vi "Get Data String.vi"(8 "error in (no error)":errorcluster, 11 "Data Cluster Out":T1 {"VestaTemperature"."Water Heater Temp (°F)" min=32 max=203}) -> (0 "error out":errorcluster, 3 "Data Cluster Output":T1={"Vesta Data Output"={"Temp_W_Raw_U"=0, "Temp_W_Raw_L"=0, "Temperature Water (F)"=0.0, "Temperature Water Compensated (F)"=0.0, "Temperature Ambient (F)"=0.0, "Setpoint Location (F)"=0.0, "Heat Request"="", "Fault Ram"="", "PWM DCDC Value"=0, "Pilot Voltage (mV)"=0.0, "Setpoint Actual (F)"=0.0, "Differential Actual (F)"=0.0, "Setpoint User (F)"=0.0, "Differential User (F)"=0.0, "Termperature FIltered -TCO (F)"=0.0, "Temp_C_Raw_1 - Sensor Voltage"="", "Temp_C_Raw_2 - Sensor Voltage"="", "Chamber Sensor Temperature (F)"=0.0, "LDO Base Temperature (F)"=0.0, "LDO Timer (sec)"=0, "Disabled (0)"=FALSE, "Warming (1)"=FALSE, "Heating (2)"=FALSE, "Cooling Data Write (3)"=FALSE, "Cooling (4)"=FALSE, "Data Read (5)"=FALSE, "N/A"=FALSE, "Temperature Trip (7)"=FALSE, "Burner"=FALSE}, "VestaTemperature"={"Water Heater Temp (°F)"=135, "Differential  (°F)"=10.0}, "Timer Application Data"={"Duty Cycle"={"Burner ON Time (Seconds)"=60.0, "Burner OFF Time (Seconds)"=60.0, "Main Burner Flag"=FALSE, "Burner Power Mode"=0}}, "Data Array"=[], "MW Output"={"TC1-Channel 021"=0.0, "TC2-Channel 022"=0.0, "TC3-Channel 023"=0.0, "TC4-Channel 024"=0.0, "TC5-Channel 025"=0.0, "TC6-Channel 026"=0.0, "TC7-Channel 017"=0.0, "TC8-Channel 028"=0.0, "TC9-Channel 029"=0.0, "TC10-Channel 030"=0.0, "TC Tree Average"=0.0, "TC DWN- Channel 027"=0.0, "RTDin-Channel 031"=0.0, "RTDout-Channel 032"=0.0, "RTDamb-Channel 033"=0.0, "PSI1-Channel 011"=0.0, "PSI2-Channel 012"=0.0, "PSI3-Channel 013"=0.0, "PSI4-Channel 014"=0.0, "UE State-Channel 015"=0.0, "LE State-Channel 016"=0.0, "Module 4 Relay Status Output"={"INTELLIFAUCET TEMP(T)/FLOW(F) (CH 041)"=FALSE, "INTELLIFAUCET READY (CH 042)"=FALSE, "INTELLIFAUCET START (CH 043)"=FALSE, "INTELLIFAUCET STOP (CH 044)"=FALSE, "MAIN POWER RELAY (CH 047)"=FALSE, "NOT USED (CH 045)"=FALSE, "NOT USED (CH 046)"=FALSE, "PURGE VALVE RELAY (CH 048)"=FALSE, "OUTLET VALVE RELAY (CH 049)"=FALSE, "INLET VALVE RELAY (CH 050)"=FALSE, "Intellifaucet (% Open)"=0.0, "Proportioning Valve (%Open)"=0.0, "Intellifaucet Temp Setpoint (F)"=0.0}}} {"VestaTemperature"."Water Heater Temp (°F)" min=32 max=203})   [LabVIEW 2023]
uses:
  controls/UI Data.ctl
  Drivers/Resideo Gas Valve/Type Definitions/Vesta Info.ctl
  Drivers/Resideo Gas Valve/Type Definitions/Temperature Control.ctl
  controls/Timer Application Cluster.ctl
  controls/Burner Duty Cycle.ctl
  Hybrid Water Heater/Type Definitions/HEWH MW100 Data Cluster.ctl
  Hybrid Water Heater/Custom Instrument Control/MW100/Type Definitions/HEWH Module 4 Relay Status.ctl
panel:
  out "Data Array":string[][](array[string])
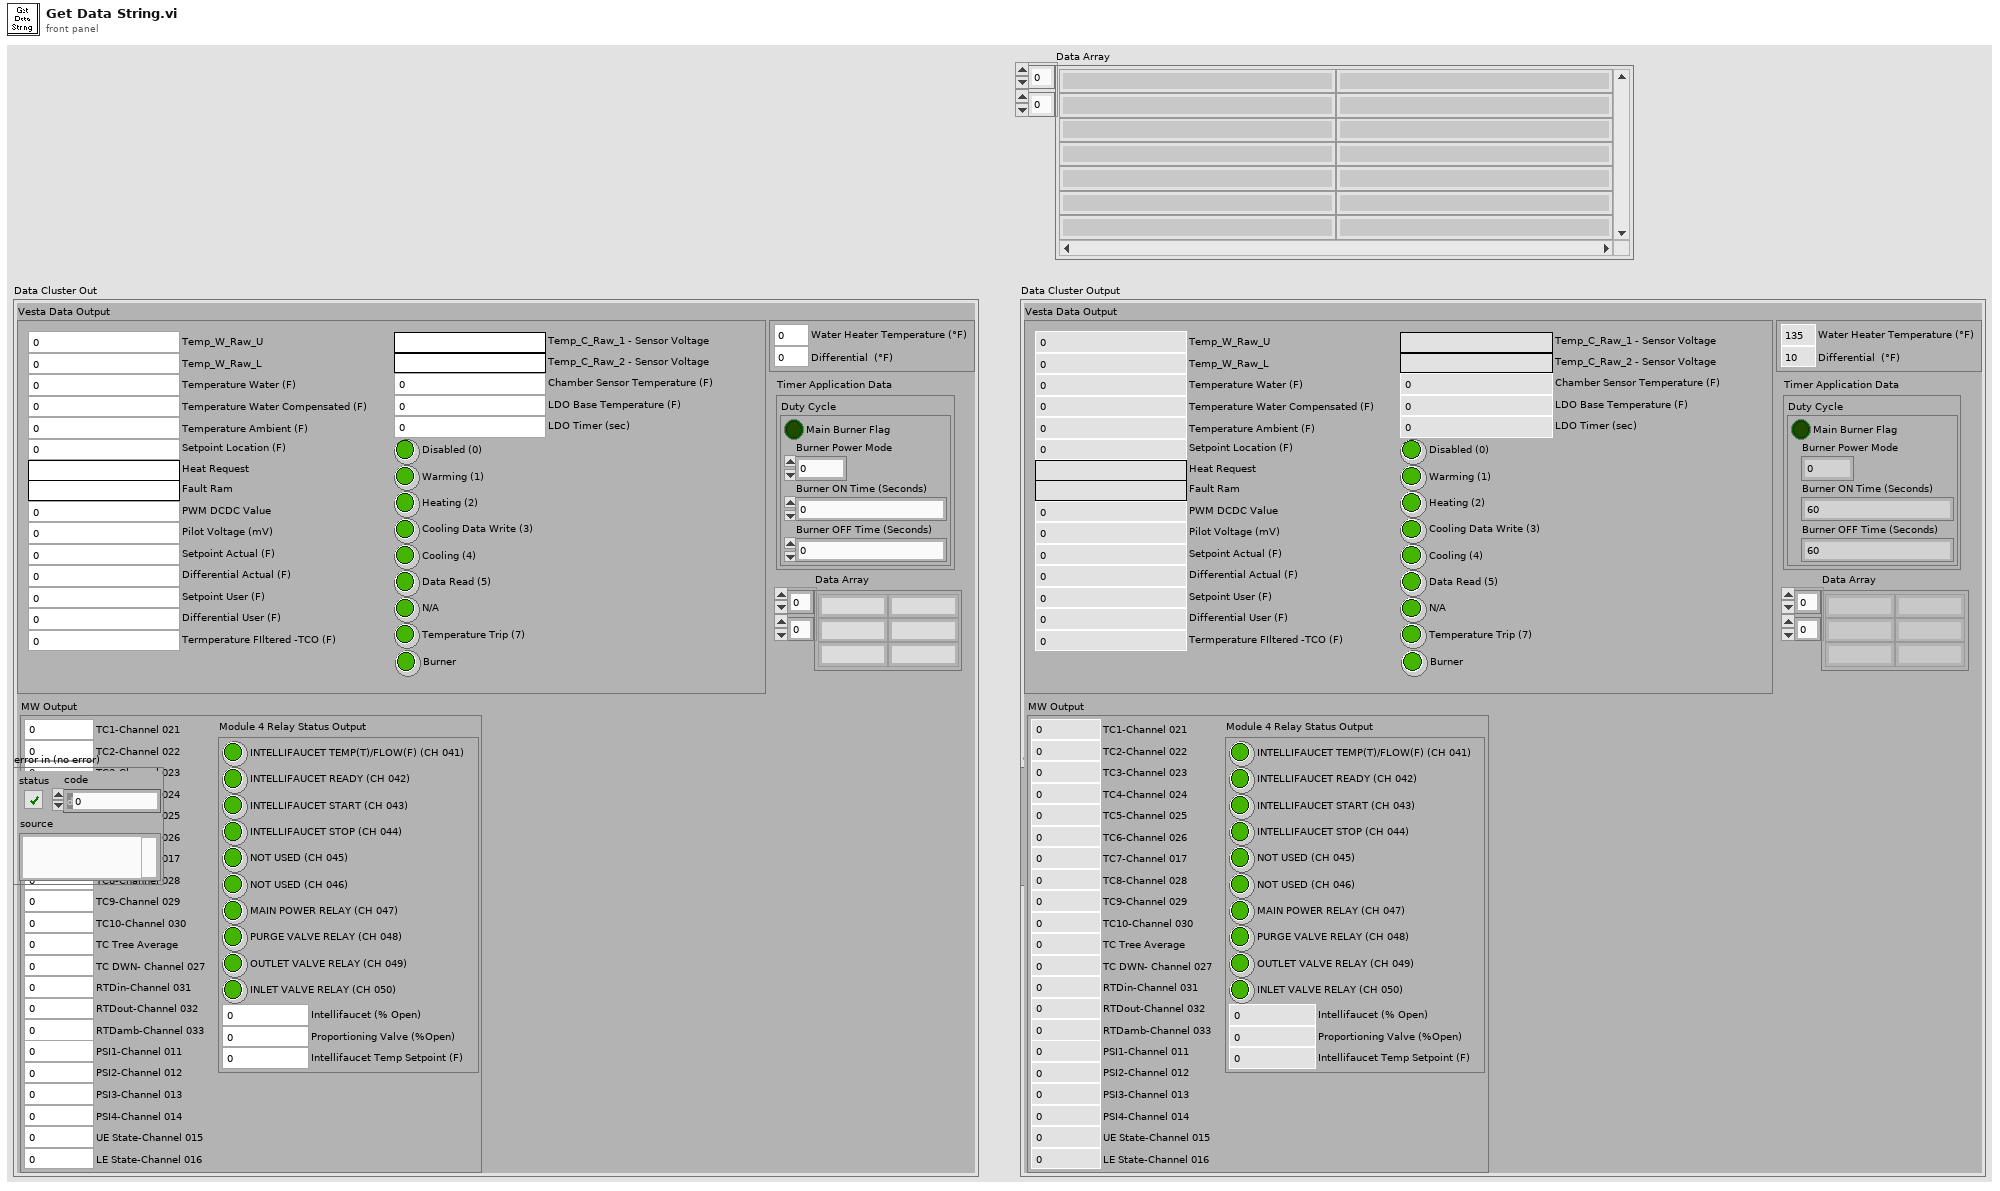
[diagram p1: front panel]
types:
  T1 = typedef "UI Data.ctl" = cluster{"Vesta Data Output":T2, "VestaTemperature":T3, "Timer Application Data":T4, "Data Array":string[][], "MW Output":T6}
  T2 = typedef "Vesta Info.ctl" = cluster{"Temp_W_Raw_U":u16, "Temp_W_Raw_L":u16, "Temperature Water (F)":dbl, "Temperature Water Compensated (F)":dbl, "Temperature Ambient (F)":dbl, "Setpoint Location (F)":dbl, "Heat Request":string, "Fault Ram":string, "PWM DCDC Value":u16, "Pilot Voltage (mV)":dbl, "Setpoint Actual (F)":dbl, "Differential Actual (F)":dbl, "Setpoint User (F)":dbl, "Differential User (F)":dbl, "Termperature FIltered -TCO (F)":dbl, "Temp_C_Raw_1 - Sensor Voltage":string, "Temp_C_Raw_2 - Sensor Voltage":string, "Chamber Sensor Temperature (F)":dbl, "LDO Base Temperature (F)":dbl, "LDO Timer (sec)":i16, "Disabled (0)":bool, "Warming (1)":bool, "Heating (2)":bool, "Cooling Data Write (3)":bool, "Cooling (4)":bool, "Data Read (5)":bool, "N/A":bool, "Temperature Trip (7)":bool, "Burner":bool}
  T3 = typedef "Temperature Control.ctl" = cluster{"Water Heater Temp (°F)":u16, "Differential  (°F)":dbl}
  T4 = typedef "Timer Application Cluster.ctl" = cluster{"Duty Cycle":T5}
  T5 = typedef "Burner Duty Cycle.ctl" = cluster{"Burner ON Time (Seconds)":dbl, "Burner OFF Time (Seconds)":dbl, "Main Burner Flag":bool, "Burner Power Mode":u8}
  T6 = typedef "HEWH MW100 Data Cluster.ctl" = cluster{"TC1-Channel 021":dbl, "TC2-Channel 022":dbl, "TC3-Channel 023":dbl, "TC4-Channel 024":dbl, "TC5-Channel 025":dbl, "TC6-Channel 026":dbl, "TC7-Channel 017":dbl, "TC8-Channel 028":dbl, "TC9-Channel 029":dbl, "TC10-Channel 030":dbl, "TC Tree Average":dbl, "TC DWN- Channel 027":dbl, "RTDin-Channel 031":dbl, "RTDout-Channel 032":dbl, "RTDamb-Channel 033":dbl, "PSI1-Channel 011":dbl, "PSI2-Channel 012":dbl, "PSI3-Channel 013":dbl, "PSI4-Channel 014":dbl, "UE State-Channel 015":dbl, "LE State-Channel 016":dbl, "Module 4 Relay Status Output":T7}
  T7 = typedef "HEWH Module 4 Relay Status.ctl" = cluster{"INTELLIFAUCET TEMP(T)/FLOW(F) (CH 041)":bool, "INTELLIFAUCET READY (CH 042)":bool, "INTELLIFAUCET START (CH 043)":bool, "INTELLIFAUCET STOP (CH 044)":bool, "MAIN POWER RELAY (CH 047)":bool, "NOT USED (CH 045)":bool, "NOT USED (CH 046)":bool, "PURGE VALVE RELAY (CH 048)":bool, "OUTLET VALVE RELAY (CH 049)":bool, "INLET VALVE RELAY (CH 050)":bool, "Intellifaucet (% Open)":dbl, "Proportioning Valve (%Open)":dbl, "Intellifaucet Temp Setpoint (F)":dbl}
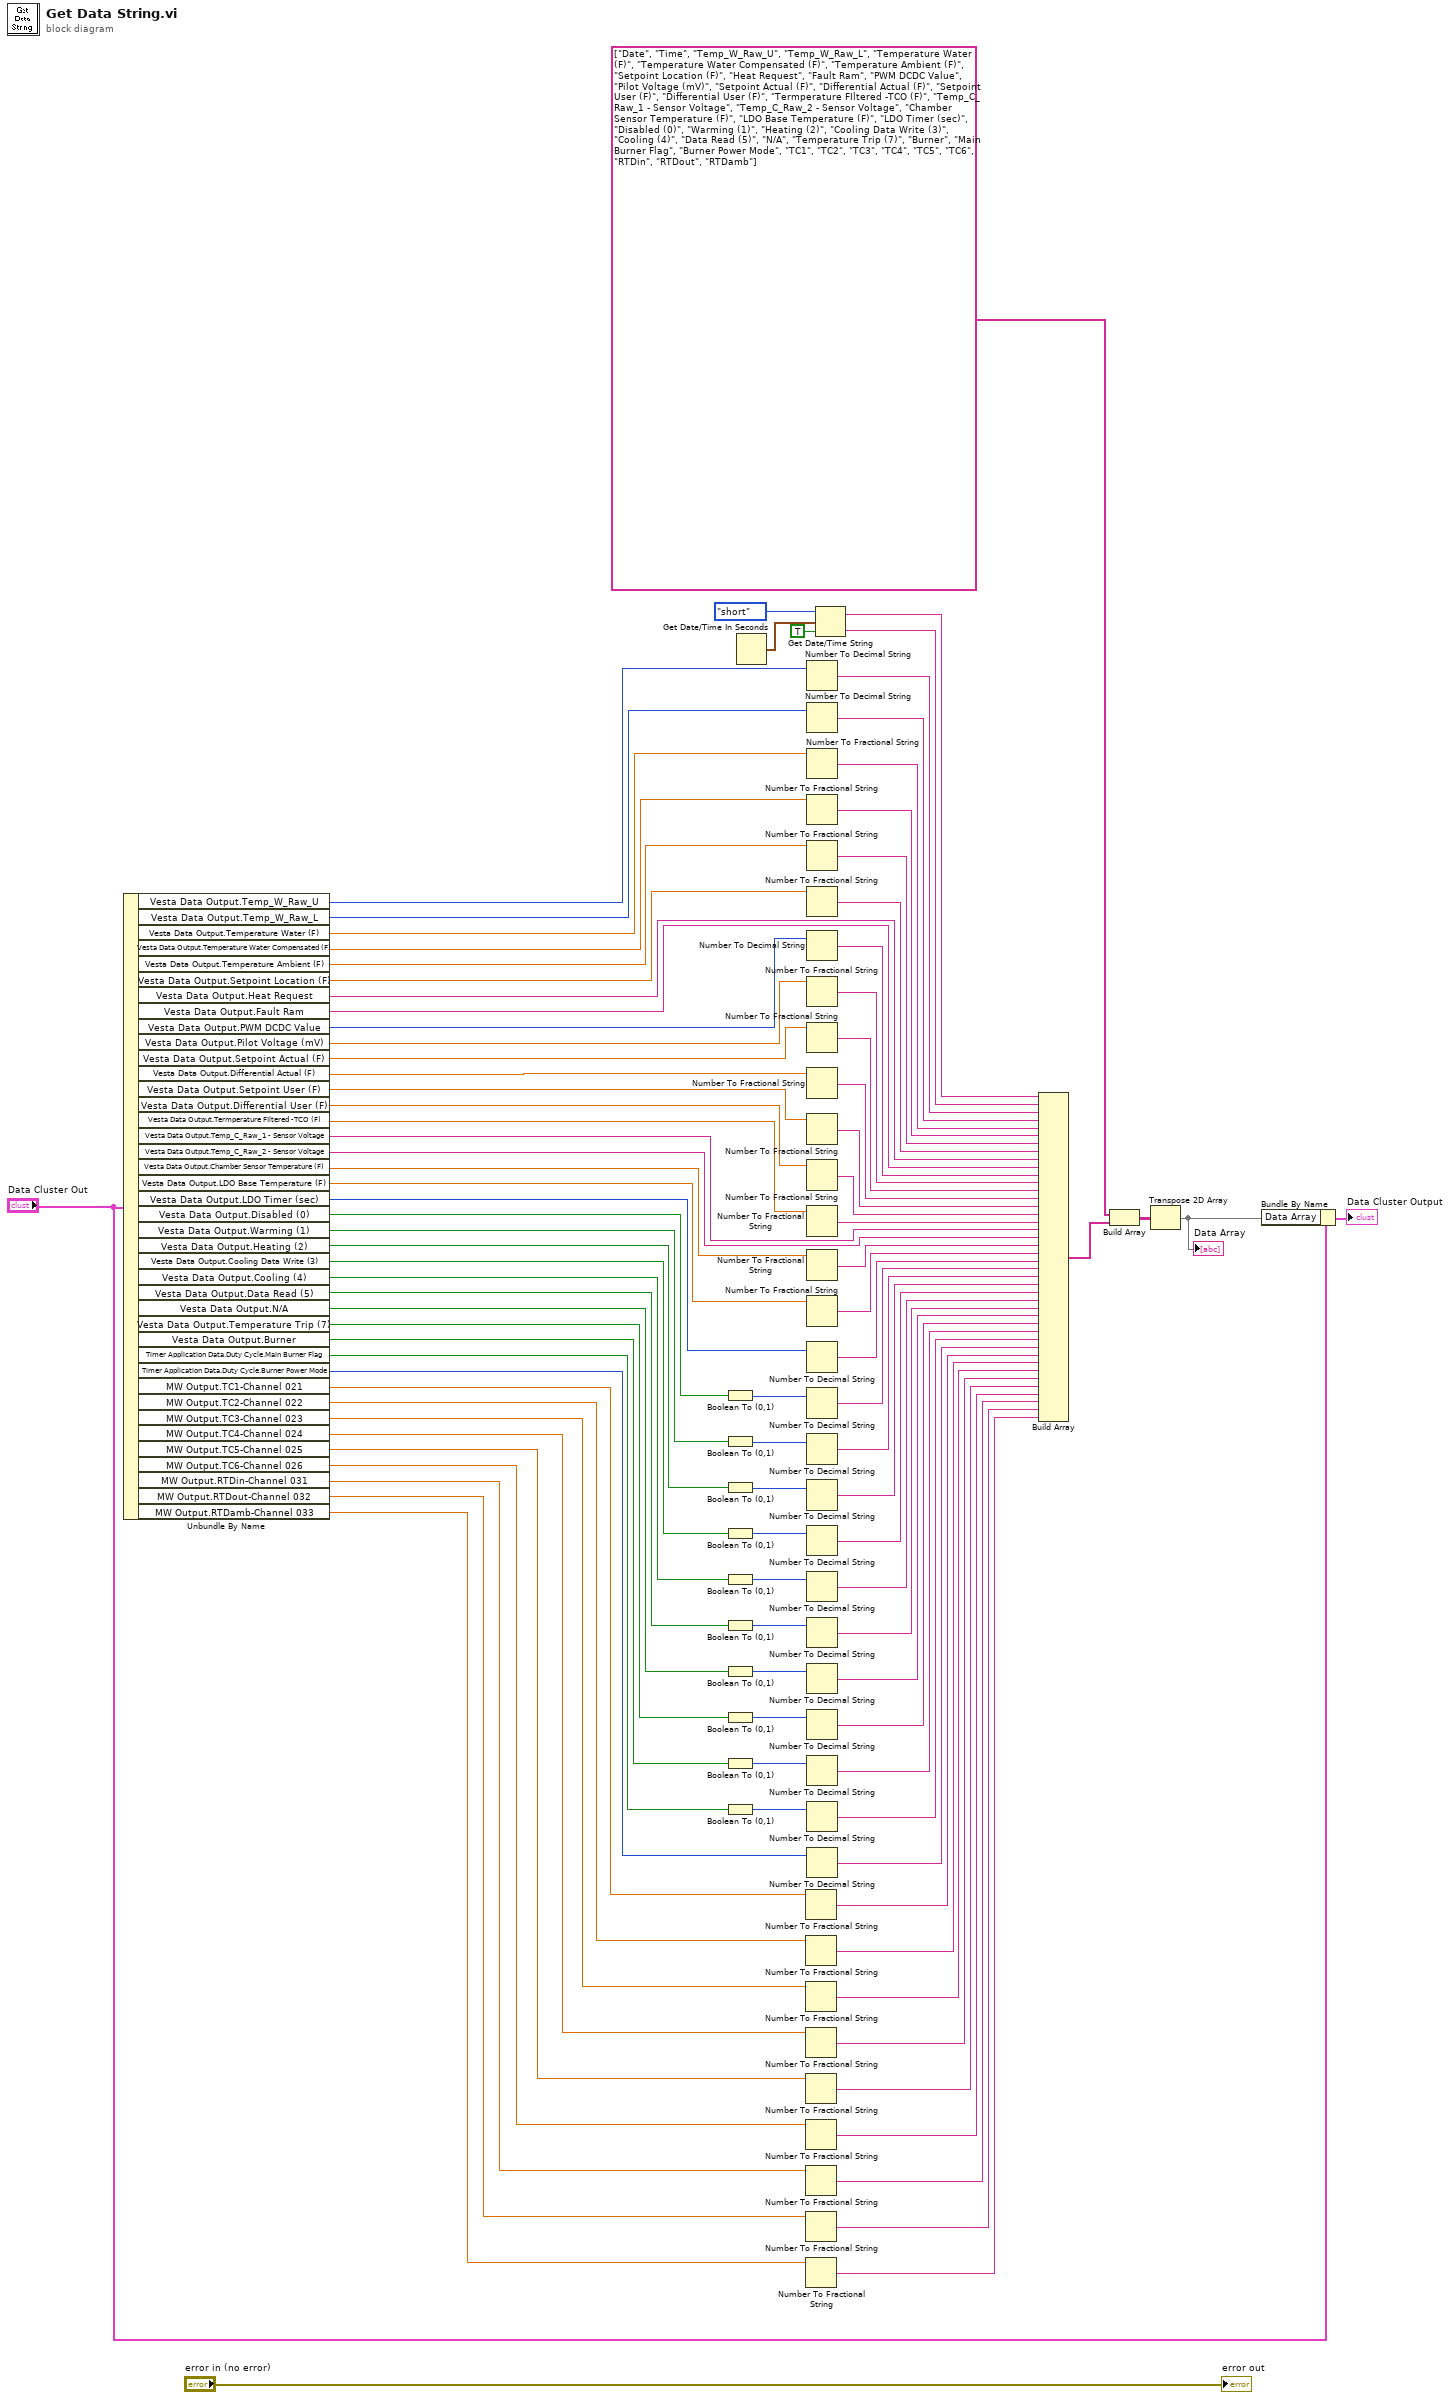
[diagram p0: block diagram]
diagram:
  n1 = Unbundle By Name("Data Cluster Out") -> ("Vesta Data Output.Temp_W_Raw_U"=w97:u16, "Vesta Data Output.Temp_W_Raw_L"=w95:u16, "Vesta Data Output.Temperature Water (F)"=w93:dbl, "Vesta Data Output.Temperature Water Compensated (F)"=w91:dbl, "Vesta Data Output.Temperature Ambient (F)"=w90:dbl, "Vesta Data Output.Setpoint Location (F)"=w89:dbl, "Vesta Data Output.Heat Request"=w85:string, "Vesta Data Output.Fault Ram"=w84:string, "Vesta Data Output.PWM DCDC Value"=w83:u16, "Vesta Data Output.Pilot Voltage (mV)"=w81:dbl, "Vesta Data Output.Setpoint Actual (F)"=w79:dbl, "Vesta Data Output.Differential Actual (F)"=w77:dbl, "Vesta Data Output.Setpoint User (F)"=w75:dbl, "Vesta Data Output.Differential User (F)"=w73:dbl, "Vesta Data Output.Termperature FIltered -TCO (F)"=w71:dbl, "Vesta Data Output.Temp_C_Raw_1 - Sensor Voltage"=w69:string, "Vesta Data Output.Temp_C_Raw_2 - Sensor Voltage"=w68:string, "Vesta Data Output.Chamber Sensor Temperature (F)"=w67:dbl, "Vesta Data Output.LDO Base Temperature (F)"=w65:dbl, "Vesta Data Output.LDO Timer (sec)"=w63:i16, "Vesta Data Output.Disabled (0)"=w60:bool, "Vesta Data Output.Warming (1)"=w57:bool, "Vesta Data Output.Heating (2)"=w54:bool, "Vesta Data Output.Cooling Data Write (3)"=w51:bool, "Vesta Data Output.Cooling (4)"=w48:bool, "Vesta Data Output.Data Read (5)"=w45:bool, "Vesta Data Output.N/A"=w42:bool, "Vesta Data Output.Temperature Trip (7)"=w39:bool, "Vesta Data Output.Burner"=w36:bool, "Timer Application Data.Duty Cycle.Main Burner Flag"=w33:bool, "Timer Application Data.Duty Cycle.Burner Power Mode"=w31:u8, "MW Output.TC1-Channel 021"=w18:dbl, "MW Output.TC2-Channel 022"=w17:dbl, "MW Output.TC3-Channel 023"=w16:dbl, "MW Output.TC4-Channel 024"=w15:dbl, "MW Output.TC5-Channel 025"=w14:dbl, "MW Output.TC6-Channel 026"=w13:dbl, "MW Output.RTDin-Channel 031"=w12:dbl, "MW Output.RTDout-Channel 032"=w11:dbl, "MW Output.RTDamb-Channel 033"=w10:dbl)
  n2 = Boolean To (0,1)(Boolean=w60) -> (0, 1=w61:i16)
  n3 = Boolean To (0,1)(Boolean=w57) -> (0, 1=w58:i16)
  n4 = Boolean To (0,1)(Boolean=w54) -> (0, 1=w55:i16)
  n5 = Boolean To (0,1)(Boolean=w51) -> (0, 1=w52:i16)
  n6 = Boolean To (0,1)(Boolean=w48) -> (0, 1=w49:i16)
  n7 = Boolean To (0,1)(Boolean=w45) -> (0, 1=w46:i16)
  n8 = Boolean To (0,1)(Boolean=w42) -> (0, 1=w43:i16)
  n9 = Boolean To (0,1)(Boolean=w39) -> (0, 1=w40:i16)
  n10 = Boolean To (0,1)(Boolean=w36) -> (0, 1=w37:i16)
  n11 = Boolean To (0,1)(Boolean=w33) -> (0, 1=w34:i16)
  n12 = Get Date/Time In Seconds() -> (seconds since 1Jan1904=w26:timestamp)
  n13 = Number To Fractional String(number=w18) -> (F-format string=w9:string)  [unwired: 3 in]
  n14 = Number To Fractional String(number=w17) -> (F-format string=w8:string)  [unwired: 3 in]
  n15 = Number To Fractional String(number=w16) -> (F-format string=w7:string)  [unwired: 3 in]
  n16 = Number To Fractional String(number=w15) -> (F-format string=w6:string)  [unwired: 3 in]
  n17 = Number To Fractional String(number=w14) -> (F-format string=w5:string)  [unwired: 3 in]
  n18 = Number To Fractional String(number=w13) -> (F-format string=w4:string)  [unwired: 3 in]
  n19 = Number To Fractional String(number=w12) -> (F-format string=w3:string)  [unwired: 3 in]
  n20 = Number To Fractional String(number=w11) -> (F-format string=w2:string)  [unwired: 3 in]
  n21 = Number To Fractional String(number=w10) -> (F-format string=w1:string)  [unwired: 3 in]
  n22 = Number To Decimal String(number=w97) -> (decimal integer string=w96:string)  [unwired: 1 in]
  n23 = Number To Decimal String(number=w95) -> (decimal integer string=w94:string)  [unwired: 1 in]
  n24 = Number To Fractional String(number=w93) -> (F-format string=w92:string)  [unwired: 3 in]
  n25 = Number To Fractional String(number=w91) -> (F-format string=w88:string)  [unwired: 3 in]
  n26 = Number To Fractional String(number=w90) -> (F-format string=w87:string)  [unwired: 3 in]
  n27 = Number To Fractional String(number=w89) -> (F-format string=w86:string)  [unwired: 3 in]
  n28 = Number To Decimal String(number=w83) -> (decimal integer string=w82:string)  [unwired: 1 in]
  n29 = Number To Fractional String(number=w81) -> (F-format string=w80:string)  [unwired: 3 in]
  n30 = Number To Fractional String(number=w79) -> (F-format string=w78:string)  [unwired: 3 in]
  n31 = Number To Fractional String(number=w77) -> (F-format string=w76:string)  [unwired: 3 in]
  n32 = Number To Fractional String(number=w75) -> (F-format string=w74:string)  [unwired: 3 in]
  n33 = Number To Fractional String(number=w73) -> (F-format string=w72:string)  [unwired: 3 in]
  n34 = Number To Fractional String(number=w71) -> (F-format string=w70:string)  [unwired: 3 in]
  n35 = Number To Fractional String(number=w67) -> (F-format string=w66:string)  [unwired: 3 in]
  n36 = Number To Fractional String(number=w65) -> (F-format string=w64:string)  [unwired: 3 in]
  n37 = Number To Decimal String(number=w63) -> (decimal integer string=w62:string)  [unwired: 1 in]
  n38 = Number To Decimal String(number=w61) -> (decimal integer string=w59:string)  [unwired: 1 in]
  n39 = Number To Decimal String(number=w58) -> (decimal integer string=w56:string)  [unwired: 1 in]
  n40 = Number To Decimal String(number=w55) -> (decimal integer string=w53:string)  [unwired: 1 in]
  n41 = Number To Decimal String(number=w52) -> (decimal integer string=w50:string)  [unwired: 1 in]
  n42 = Number To Decimal String(number=w49) -> (decimal integer string=w47:string)  [unwired: 1 in]
  n43 = Number To Decimal String(number=w46) -> (decimal integer string=w44:string)  [unwired: 1 in]
  n44 = Number To Decimal String(number=w43) -> (decimal integer string=w41:string)  [unwired: 1 in]
  n45 = Number To Decimal String(number=w40) -> (decimal integer string=w38:string)  [unwired: 1 in]
  n46 = Number To Decimal String(number=w37) -> (decimal integer string=w35:string)  [unwired: 1 in]
  n47 = Number To Decimal String(number=w34) -> (decimal integer string=w32:string)  [unwired: 1 in]
  n48 = Number To Decimal String(number=w31) -> (decimal integer string=w30:string)  [unwired: 1 in]
  n49 = Get Date/Time String(date format (0)=enum16{"short", "long", "abbreviated"}."short", seconds (now)=w26, want seconds? (F)=TRUE) -> (date string=w24:string, time string=w23:string)
  n50 = Build Array(w24, w23, w96, w94, w92, w88, w87, w86, w85, w84, w82, w80, w78, w76, w74, w72, w70, w69, w68, w66, w64, w62, w59, w56, w53, w50, w47, w44, w41, w38, w35, w32, w30, w9, w8, w7, w6, w5, w4, w3, w2, w1) -> (w28:string[])
  n51 = Build Array(string[] ["Date", "Time", "Temp_W_Raw_U", "Temp_W_Raw_L", "Temperature Water (F)", "Temperature Water Compensated (F)", "Temperature Ambient (F)", "Setpoint Location (F)", "Heat Request", "Fault Ram", "PWM DCDC Value", "Pilot Voltage (mV)", "Setpoint Actual (F)", "Differential Actual (F)", "Setpoint User (F)", "Differential User (F)", "Termperature FIltered -TCO (F)", "Temp_C_Raw_1 - Sensor Voltage", "Temp_C_Raw_2 - Sensor Voltage", "Chamber Sensor Temperature (F)", "LDO Base Temperature (F)", "LDO Timer (sec)", "Disabled (0)", "Warming (1)", "Heating (2)", "Cooling Data Write (3)", "Cooling (4)", "Data Read (5)", "N/A", "Temperature Trip (7)", "Burner", "Main Burner Flag", "Burner Power Mode", "TC1", "TC2", "TC3", "TC4", "TC5", "TC6", "RTDin", "RTDout", "RTDamb"], w28) -> (w27:string[][])
  n52 = Transpose 2D Array(2D array=w27) -> (transposed array=w19:string[][])
  "Data Array" <- w19
  n53 = Bundle By Name(cluster="Data Cluster Out", "Data Array"=w19) -> (→"Data Cluster Output":T1)
  "error out" <- "error in (no error)"
